vi "P1v2.vi"() -> ()   [LabVIEW 2017]
uses:
  <vilib>/sound2/lvsound2.llb/Sampling Mode.ctl
  <vilib>/sound2/lvsound2.llb/Sound Data Format.ctl
  <vilib>/Analysis/2dsp.llb/Inverse Real FFT.vi
  <vilib>/ptbypt/Frequency Domain.llb/Real FFT PtByPt.vi
  <vilib>/sound2/lvsound2.llb/Sound Input Read (DBL).vi
  <vilib>/express/express analysis/Spectral/Block/exnSpectralBlock spectral measurements power poly.vi
  <vilib>/express/express analysis/Spectral/Block/exnSpectralBlock spectral measurements power WFM.vi
  <vilib>/measure/mamon.llb/Waveform Peak Detection for 1 Chan.vi
  <vilib>/express/express analysis/Spectral/Block/exnSpectralBlock spectral measurements peak poly.vi
  <vilib>/express/express analysis/Spectral/Block/exnSpectralBlock spectral measurements peak WFM.vi
  <vilib>/express/express analysis/Spectral/XNode/ExpressSpectralMeasurementsBlockNode.xnode
  <vilib>/measure/NI_MAPro.lvlib
  <vilib>/ptbypt/NI_PtbyPt.lvlib
  <vilib>/Analysis/NI_AALPro.lvlib
panel:
  out "convolucion":dbl[](graph)
  in  "Sensitivity":dbl(slide)=10.0 scale=1.0..100.0
  out "Peak Locations":dbl[](array[numeric]) format="%#.1f"
  out "System Intensity Chart":dbl[][](graph)
  out "Frequency Power Spectrum":cluster{"f0":dbl, "df":dbl, "magnitude":dbl[]}(graph)
  out "Time domain signal":waveform(dbl)(graph)
  in  "stop":bool
  # "PROYECTO D"
  # "IDENTIFICACIÓN DE COMPONENTES ARMÓNICAS EN UNA SEÑAL DE AUDIO"
  # "Entrada de la señal de audio"
  # "Correspondiente en el dominio de la frecuencia de la señal de audio"
  # "Convolución de la señal recibida con una de tipo diente de sierra"
  # "Espectrograma que muestra la evolución temporal de las componentes de frecuencia"
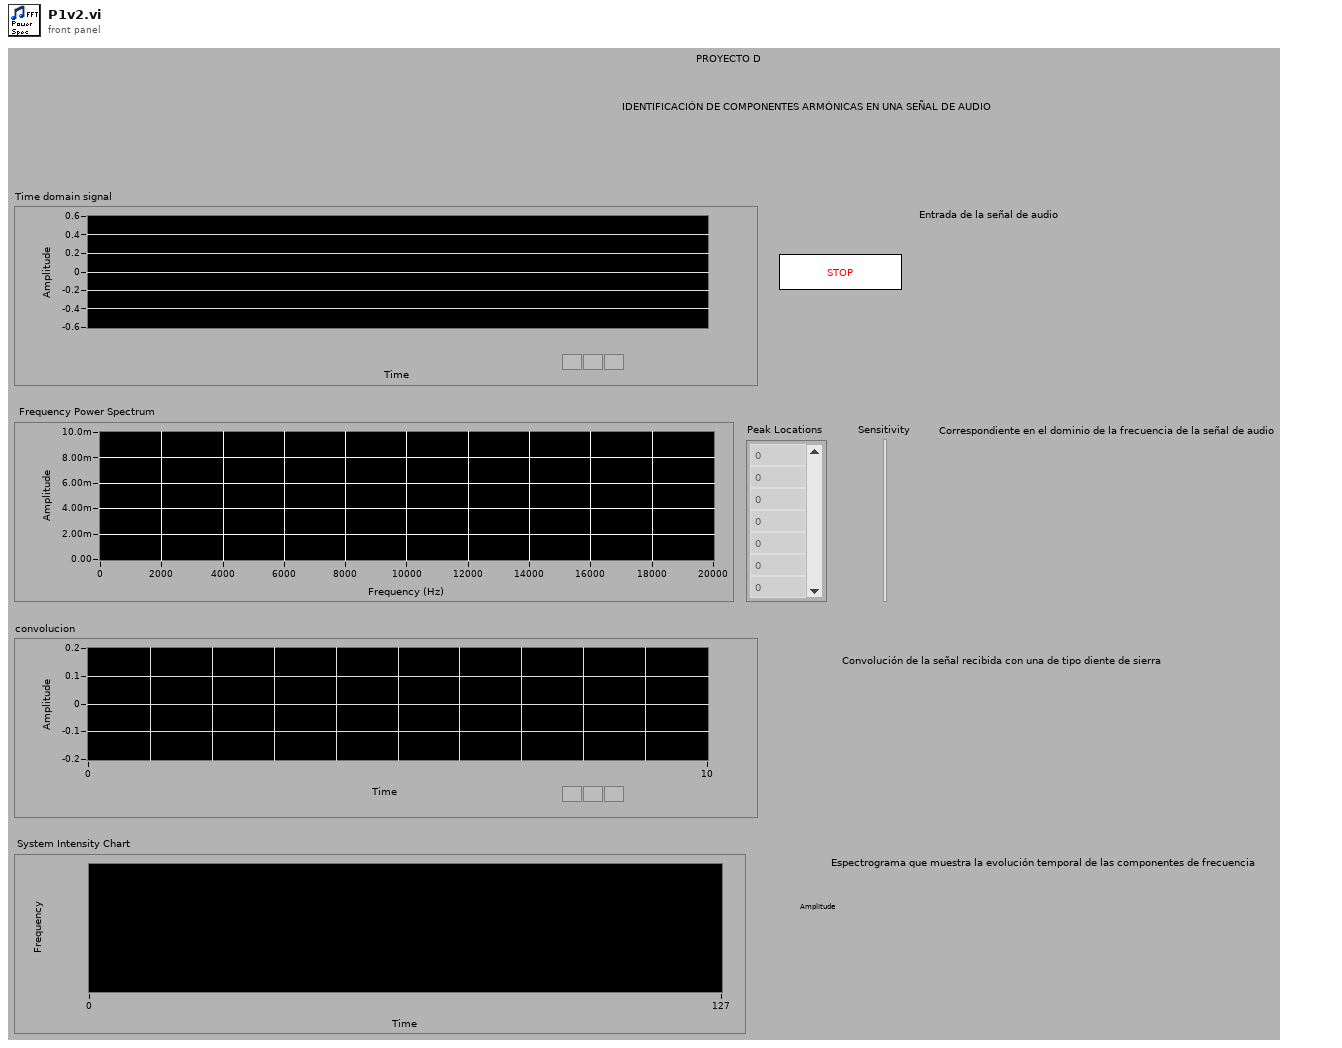
[diagram p1: front panel]
types:
  T1 = typedef "Sound Data Format.ctl" = cluster{"sample rate (S/s)":dbl, "number of channels":i32, "bits per sample":i32}
  T2 = typedef "Sampling Mode.ctl" = i32
  T3 = typedef "Sound Input Task ID.ctl" = u32
  T4 = cluster{"averaging mode":u16, "weighting mode":u16, "number of averages":u32}
  T5 = cluster{"dB On (F)":bool, "unwrap phase (F)":bool, "convert to degree (F)":bool}
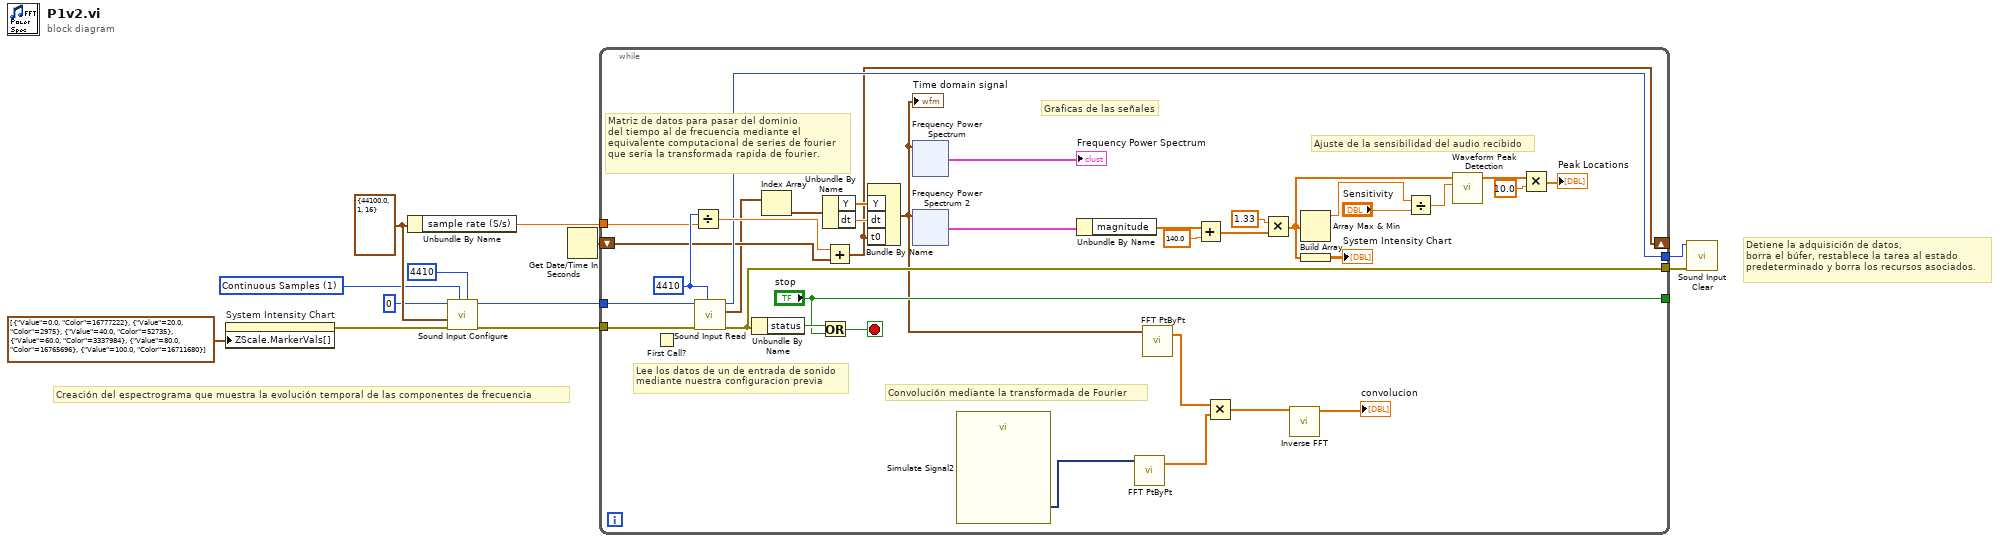
[diagram p0: block diagram]
diagram:
  w11 = T1 {"sample rate (S/s)"=44100.0, "number of channels"=1, "bits per sample"=16} ("sound format")
  w9 = T2 1 items=["Finite Samples", "Continuous Samples"] ("sample mode")
  # "Creación del espectrograma que muestra la evolución temporal de las componentes de frecuencia"
  # "Detiene la adquisición de datos,\nborra el búfer, restablece la tarea al estado\npredeterminado y borra los recursos asociados."
  n1 = property on="System Intensity Chart" class="IntChart (strict)"("ZScale.MarkerVals[]"=cluster{"Value":dbl, "Color":u32}[] [{"Value"=0.0, "Color"=16777222}, {"Value"=20.0, "Color"=2975}, {"Value"=40.0, "Color"=52735}, {"Value"=60.0, "Color"=3337984}, {"Value"=80.0, "Color"=16765696}, {"Value"=100.0, "Color"=16711680}]) -> (error out=w2:errorcluster)  [unwired: 2 in, 1 out]
  n2 = Unbundle By Name(w11) -> ("sample rate (S/s)"=w12:dbl)
  n3 = call <vilib>:"Sound Input Configure.vi"("number of samples/ch"=4410 ("Number of Samples"), "sample mode"=w9, "error in (no error)"=w2, "sound format"=w11, "device ID"=u32 0) -> ("error out"=w6:errorcluster, "task ID"=w5:T3)  [unwired: 5 in]
  n4 = Get Date/Time In Seconds() -> (seconds since 1Jan1904=w4:timestamp)
  n5 = while {
    tunnel: w6 -> [w48]
    tunnel: w12 -> [w43]
    tunnel: [w41] -> w7
    tunnel: w5 -> [w40]
    tunnel: [w39] -> w8
    shift-right: [w21] -> _
    shift-left: w4 -> [w38]
    tunnel: ["stop"] -> _
    stop <- w36 stop-if-true
    w44 = 4410 ("Number of samples\n per Read")
    # "Ajuste de la sensibilidad del audio recibido"
    # "Matriz de datos para pasar del dominio\ndel tiempo al de frecuencia mediante el\nequivalente computacional de series de fourier\nque seria la transformada rapida de fourier."
    # "Graficas de las señales"
    # "Lee los datos de un de entrada de sonido\nmediante nuestra configuracion previa"
    # "Convolución mediante la transformada de Fourier"
    n6 = First Call?() -> ()  [unwired: 1 out]
    n7 = Divide(x=w44, y=w43) -> (x/y=w42:dbl)
    n8 = call-poly <vilib>:"Sound Input Read.vi"("number of samples/ch"=w44, "error in (no error)"=w48, "task ID"=w40) -> ("error out"=w41:errorcluster, "data"=w22:waveform(dbl)[], "task ID out"=w39:T3)  [unwired: 6 in]
    n9 = Unbundle By Name(w41) -> ("status"=w37:bool)
    n10 = Index Array(array=w22) -> (element=w47:waveform(dbl))  [unwired: 1 in]
    n11 = Or(x=w37, y="stop") -> (x .or. y?=w36:bool)
    n12 = Unbundle By Name(w47) -> ("Y"=w46:dbl[], "dt"=w45:dbl)
    n13 = Add(x=w42, y=w38) -> (x+y=w21:timestamp)
    n14 = Bundle By Name("Y"=w46, "dt"=w45, "t0"=w21) -> (w13:waveform(dbl))  [unwired: 1 in]
    "Time domain signal" <- w13
    n15 = xnode "Frequency Power Spectrum"("Signals"=w13) -> ("FFT - (Peak)"=→"Frequency Power Spectrum":cluster{"f0":dbl, "df":dbl, "magnitude":dbl[]})  [unwired: 1 in, 2 out]
    n16 = xnode "Frequency Power Spectrum 2"("Signals"=w13) -> ("Power Spectrum"=w23:cluster{"f0":dbl, "df":dbl, "magnitude":dbl[]})  [unwired: 1 in, 1 out]
    n17 = call "Simulate Signal2"() -> ("Sawtooth"=w14:dynamicdata)  [unwired: 14 in, 1 out]
    n18 = Unbundle By Name(w23) -> ("magnitude"=w29:dbl[])
    n19 = call-poly <vilib>:"FFT PtByPt.vi"("x"=w14) -> ("FFT{X}"=w16:cdb[])  [unwired: 3 in, 1 out]
    n20 = call-poly <vilib>:"FFT PtByPt.vi"("x"=w13) -> ("FFT{X}"=w15:cdb[])  [unwired: 3 in, 1 out]
    n21 = Add(x=w29, y=140.0 ("sample rate (S/s)")) -> (x+y=w28:dbl[])
    n22 = Multiply(x=w15, y=w16) -> (x*y=w17:cdb[])
    n23 = Multiply(x=1.33 ("sample rate (S/s)"), y=w28) -> (x*y=w26:dbl[])
    n24 = call-poly <vilib>:"Inverse FFT.vi"("FFT {X}"=w17) -> ("X"=→"convolucion":dbl[])  [unwired: 9 in, 1 out]
    n25 = Array Max & Min(array=w26) -> (max value=w31:dbl)  [unwired: 3 out]
    n26 = Build Array(w26) -> (→"System Intensity Chart":dbl[][])
    n27 = Divide(x=w31, y="Sensitivity") -> (x/y=w19:dbl)
    n28 = call-poly <vilib>:"Waveform Peak Detection.vi"("threshold"=w19, "Signal In"=w26) -> ("Locations"=w33:dbl[])  [unwired: 5 in, 4 out]
    n29 = Multiply(x=w33, y=10.0 ("sample rate (S/s)")) -> (x*y=→"Peak Locations":dbl[])
  }
  n30 = call <vilib>:"Sound Input Clear.vi"("error in (no error)"=w7, "task ID"=w8) -> ()  [unwired: 9 in, 1 out]
